vi "Modified_LuaL_Buffer.vi"(11 "luaL_Buffer *B":T2) -> ()   [LabVIEW 2011]
panel:
  out "输出簇":T1
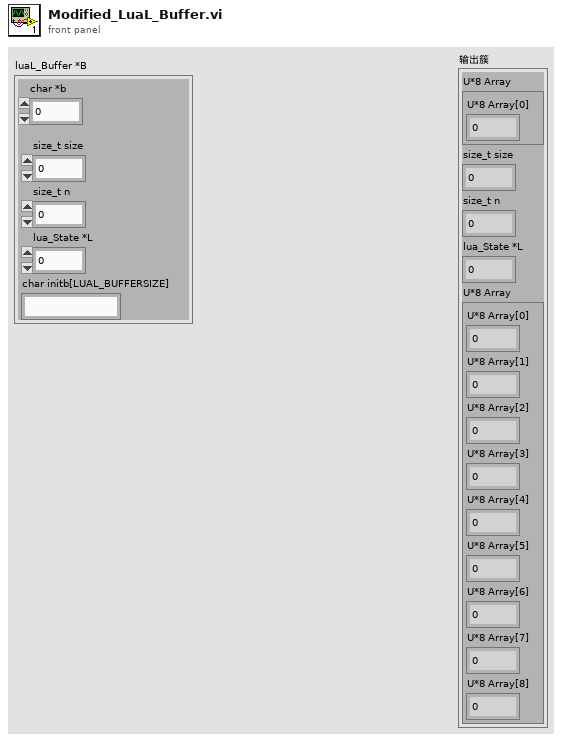
[diagram p1: front panel]
types:
  T1 = cluster{"U*8 Array":cluster{"U*8 Array[0]":u8}, "size_t size":u32, "size_t n":u32, "lua_State *L":u64, "U*8 Array":cluster{"U*8 Array[0]":u8, "U*8 Array[1]":u8, "U*8 Array[2]":u8, "U*8 Array[3]":u8, "U*8 Array[4]":u8, "U*8 Array[5]":u8, "U*8 Array[6]":u8, "U*8 Array[7]":u8, "U*8 Array[8]":u8}}
  T2 = cluster{"char *b":u64, "size_t size":u32, "size_t n":u32, "lua_State *L":u64, "char initb[LUAL_BUFFERSIZE]":string}
  T3 = cluster{"U*8 Array[0]":u8, "U*8 Array[1]":u8, "U*8 Array[2]":u8, "U*8 Array[3]":u8, "U*8 Array[4]":u8, "U*8 Array[5]":u8, "U*8 Array[6]":u8, "U*8 Array[7]":u8, "U*8 Array[8]":u8}
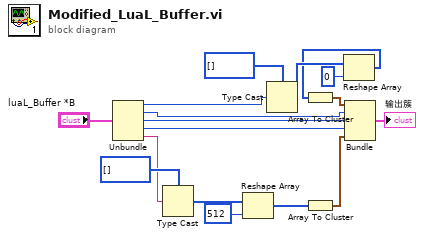
[diagram p0: block diagram]
diagram:
  n1 = Unbundle("luaL_Buffer *B") -> ("char *b"=w17:u64, "size_t size"=w11:u32, "size_t n"=w12:u32, "lua_State *L"=w13:u64, "char initb[LUAL_BUFFERSIZE]"=w14:string)
  n2 = Type Cast(type=u8[] [] ("U*8 Array"), x=w14) -> (*(type *) &x=w8:u8[])
  n3 = Reshape Array(w8, 512 ("维数大小")) -> (w5:u8[])
  n4 = Type Cast(type=u8[] [] ("U*8 Array"), x=w17) -> (*(type *) &x=w4:u8[])
  n5 = Array To Cluster(array=w5) -> (cluster=w6:T3)
  n6 = Reshape Array(w4, 0 ("维数大小")) -> (w2:u8[])
  n7 = Array To Cluster(array=w2) -> (cluster=w9:cluster{"U*8 Array[0]":u8})
  n8 = Bundle("U*8 Array"=w9, "size_t size"=w11, "size_t n"=w12, "lua_State *L"=w13, "U*8 Array"=w6) -> (→"输出簇":T1)  [unwired: 1 in]
